vi "Do.vi"(8 "error in (no error)":errorcluster, 10 "Actor in":refnum<class "Actor.lvclass">, 11 "Start Stop Scan Msg":refnum<class "Start Stop Scan Msg.lvclass">) -> (0 "error out":errorcluster, 2 "Actor out":refnum<class "Actor.lvclass">)   [LabVIEW 2013, in "Generic Data Logger.lvlib" / "Fluke 2625A (Hydra II).lvlib" / "Start Stop Scan Msg.lvclass"]
doc: "This VI delivers the message to the actor by calling the appropriate method(s) on the actor."
uses:
  Start Stop Scan Msg.lvclass
  <vilib>/ActorFramework/Actor/Actor.lvclass
  Fluke 2625A (Hydra II)/Fluke 2625A (Hydra II).lvclass
  Start Stop Scan Msg.lvclass/Start Stop Scan Msg.ctl
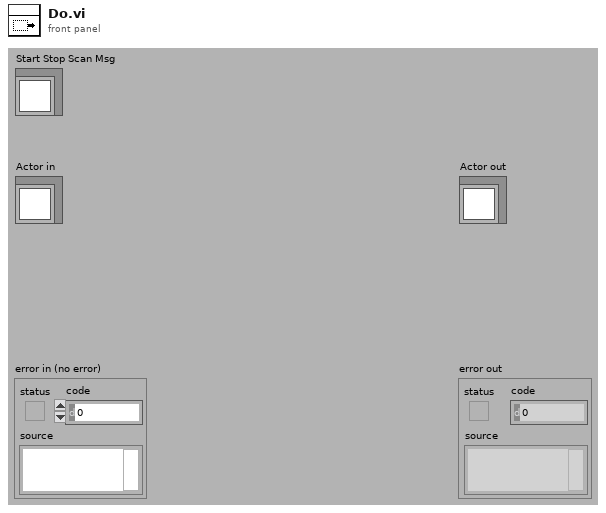
[diagram p1: front panel]
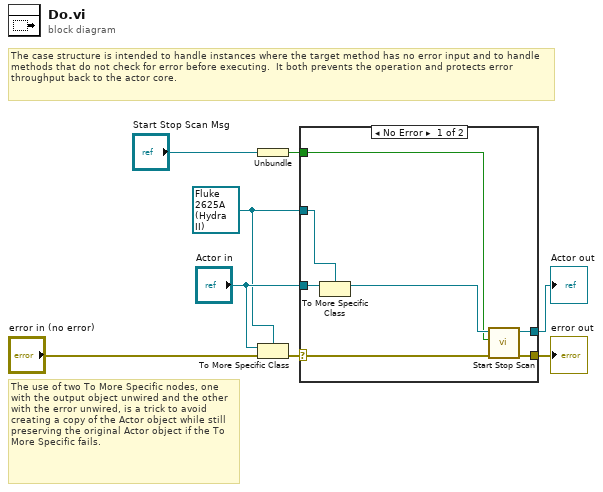
[diagram p0: block diagram]
diagram:
  w2 = refnum<class "Fluke 2625A (Hydra II).lvclass"> refnum ("Actor in")
  # "The use of two To More Specific nodes, one with the output object unwired and the other with the error unwired, is a trick to avoid creating a copy of the Actor object while still preserving the original Actor object if the To More Specific fails."
  # "The case structure is intended to handle instances where the target method has no error input and to handle methods that do not check for error before executing.  It both prevents the operation and protects error throughput back to the actor core."
  n1 = Unbundle("Start Stop Scan Msg") -> (w1:bool)
  n2 = To More Specific Class(target class=w2, reference="Actor in", error in="error in (no error)") -> (error out=w6:errorcluster)  [unwired: 1 out]
  n3 = case shown="No Error" w6 {
    selector: w6 -> [w13 w17]
    tunnel: [w15 w17] -> w5
    tunnel: [w14 w16] -> w4
    tunnel: "Actor in" -> [w12 w16]
    tunnel: w2 -> [w11 _]
    tunnel: w1 -> [w9 _]
    frame No Error {
      n4 = To More Specific Class(target class=w11, reference=w12) -> (specific class reference=w10:refnum<class "Fluke 2625A (Hydra II).lvclass">)  [unwired: 1 in, 1 out]
      n5 = call "Start Stop Scan.vi"("error in (no error)"=w13, "Start/Stop"=w9, "Generic Data Logger.lvlib:Fluke 2625A (Hydra II).lvlib:Fluke 2625A (Hydra II).lvclass"=w10) -> ("error out"=w15:errorcluster, "Generic Instrument out"=w14:refnum<class "Fluke 2625A (Hydra II).lvclass">)  [unwired: 7 in]
    }
    frame Error {
      # "If type check fails, pass the original object out again."
    }
  }
  "error out" <- w5
  "Actor out" <- w4
